vi "BW DB Path.vi"() -> (0 "DB Path":string)   [LabVIEW 2017]
doc: "Returns the path to our database."
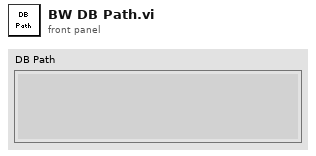
[diagram p1: front panel]
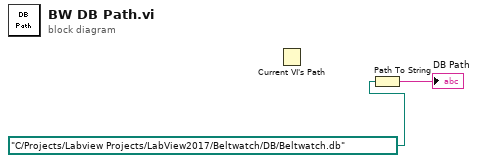
[diagram p0: block diagram]
diagram:
  n1 = Current VI's Path() -> ()  [unwired: 1 out]
  n2 = Path To String(path=path "C:/Projects/Labview Projects/LabView2017/Beltwatch/DB/Beltwatch.db" ("Path")) -> (string=→"DB Path":string)
